vi "InitialStateNode_GetClassAttributes.vi"(0 "reference in":refnum<class "InitialStateNode.lvclass">, 5 "error in (no error)":errorcluster) -> (14 "reference out":refnum<class "InitialStateNode.lvclass">, 16 "Class attributes out":T1, 17 "Attributes locked?":bool, 19 "error out":errorcluster)   [LabVIEW 2016, in "InitialStateNode.lvclass"]
doc: "Returns the class attributes of a InitialStateNode class. If reference is wired, the class attributes of the class (or sub class) will be returned else the class attributes will default to the InitialStateNode class.\n\nIf the data is currently locked for modification, 'Attributes locked?' will return TRUE. If reference is wired, the class attributes of the class (or sub class) will be returned else the class attributes of the InitialStateNode.\n\n[GOOP 2.0.15]"
uses:
  <resource>/Framework/Providers/Open_GDS/UML/InitialStateNode_class/InitialStateNode.lvclass
  <vilib>/addons/_goop3.llb/3GOOPStates.ctl
  <resource>/Framework/Providers/Open_GDS/UML/AbstractNode_class/protected/ClassAttributes.ctl
  <resource>/Framework/Providers/Open_GDS/UML/AbstractNode_class/AbstractNode.lvclass
  <resource>/Framework/Providers/Open_GDS/UML/RectangularNode_class/protected/ClassAttributes.ctl
  <resource>/Framework/Providers/Open_GDS/UML/RectangularNode_class/RectangularNode.lvclass
  <resource>/Framework/Providers/Open_GDS/UML/InitialStateNode_class/protected/ClassAttributes.ctl
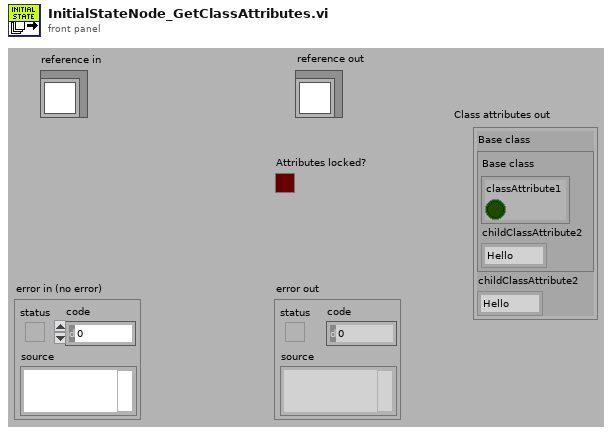
[diagram p1: front panel]
types:
  T1 = typedef "InitialStateNode.lvclass/ClassAttributes.ctl" = cluster{"Base class":T2, "childClassAttribute2":enum16{"Hello", "Goodbye"}}
  T2 = typedef "RectangularNode.lvclass/ClassAttributes.ctl" = cluster{"Base class":T3, "childClassAttribute2":enum16{"Hello", "Goodbye"}}
  T3 = typedef "AbstractNode.lvclass/ClassAttributes.ctl" = cluster{"classAttribute1":bool}
  T4 = typedef "3GOOPStates.ctl" = enum16{"Set", "Get", "New", "Delete", "Clear", "Test and get", "Unlock data", "Information", "Look up existing", "New or look up existing", "Test and get shared", "Get shared", "Set shared", "Unlock shared", "Find dynamic method", "Register dynamic method", "Preload dynamic method", "Probe", "Cast to more generic", "Cast to more specific"}
  T5 = typedef "AbstractNode.lvclass/ObjectReference.ctl" = refnum<k1>
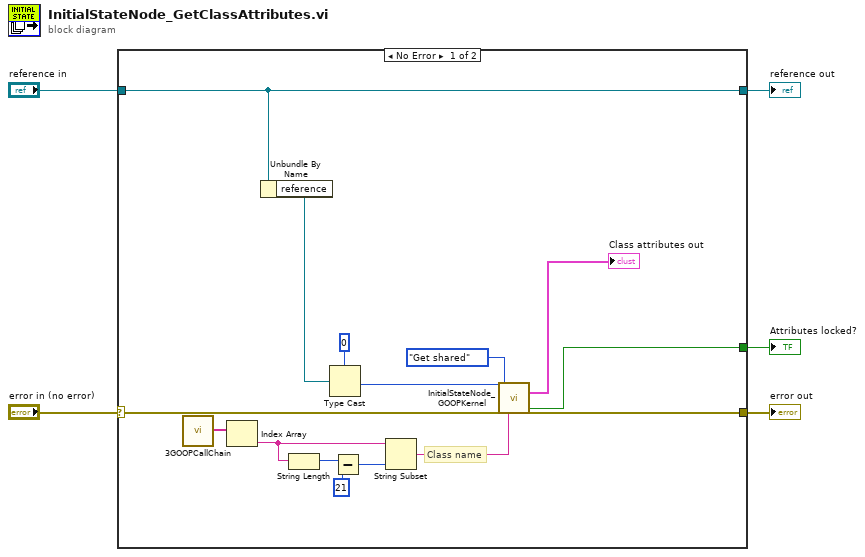
[diagram p0: block diagram]
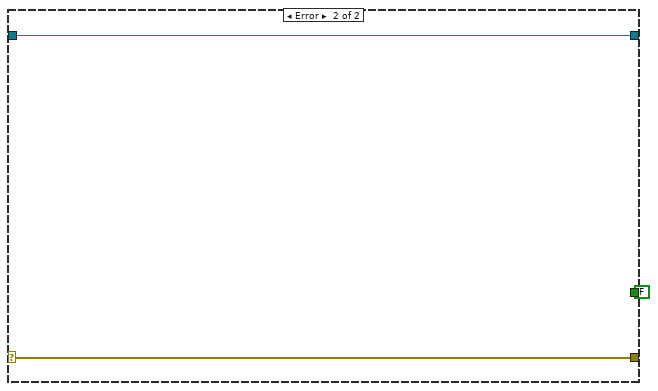
[diagram p2: hidden frame]
diagram:
  n1 = case shown="No Error" "error in (no error)" {
    selector: "error in (no error)" -> [w15 w22]
    tunnel: [w17 w23] -> w5
    tunnel: [w20 w22] -> w4
    tunnel: "reference in" -> [w17 w23]
    tunnel: [w19 FALSE ("Data locked?")] -> w1
    frame No Error {
      # "Class name"
      n2 = call <vilib>:"3GOOPCallChain.vi"() -> ("call chain"=w6:string[])
      n3 = Index Array(array=w6) -> (element=w9:string)  [unwired: 1 in]
      n4 = Unbundle By Name(w17) -> ("reference"=w7:T5)
      n5 = String Length(string=w9) -> (length=w12:i32)
      n6 = Type Cast(type=0, x=w7) -> (*(type *) &x=w18:i32)
      n7 = Subtract(x=w12, y=21) -> (x-y=w10:i32)
      n8 = String Subset(string=w9, length (rest)=w10) -> (substring=w8:string)  [unwired: 1 out]
      n9 = call <resource>:"InitialStateNode_GOOPKernel.vi"("Ref in"=w18, "error in (no error)"=w15, "Action"=3GOOPStates."Get shared", "Dynamic VI name"=w8) -> ("Data shared out"=→"Class attributes out":T1, "Data locked?"=w19:bool, "error out"=w20:errorcluster)  [unwired: 11 in, 10 out]
    }
    frame Error {
    }
  }
  "error out" <- w4
  "reference out" <- w5
  "Attributes locked?" <- w1
